vi "editConfiguration.vi"   [LabVIEW 2013]
uses:
  <userlib>/Common/ConfigurationEditor/ConfigurationEditor.lvclass
types:
  T1 = enum32{"Bad", "Idle", "Run top level", "Running"}
  T2 = enum32{"Invalid", "Standard", "Closed", "Hidden", "Minimized", "Maximized"}
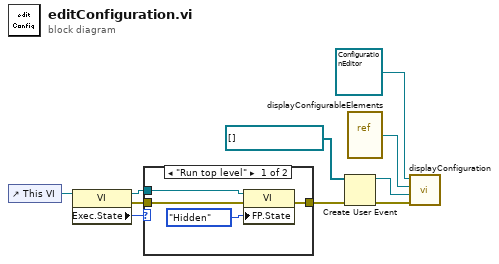
[diagram p0: block diagram]
diagram:
  n1 = control-ref of="This VI"() -> (w5:refnum<vi>)
  n2 = property class="VI"(reference=w5) -> (reference out=w3:refnum<vi>, error out=w1:errorcluster, "Exec.State"=w4:T1)  [unwired: 1 in]
  n3 = case shown="\"Run top level\"" w4 {
    tunnel: w3 -> [w13 _]
    tunnel: [w12 w15] -> w2
    tunnel: w1 -> [w11 w15]
    frame "Run top level" {
      n4 = property class="VI"(reference=w13, error in=w11, "FP.State"=T2."Hidden" ("Front Panel Window:State")) -> (error out=w12:errorcluster)  [unwired: 1 out]
    }
    frame "Running", Default {
    }
  }
  n5 = Create User Event(user event datatype=refnum<vi>[] [] ("cfgCtrlRefs"), error in=w2) -> (user event=w7:refnum<user-event>, error out=w6:errorcluster)
  n6 = vi-ref "displayConfigurableElements.vi"() -> (w10:refnum<vi>)
  n7 = call <userlib>:"displayConfiguration.vi"("error in (no error)"=w6, "ctrlRefArrayUsrEvnt"=w7, "configurableElementsVI"=w10, "ConfigurationEditor in"=refnum<class "ConfigurationEditor.lvclass"> refnum) -> ()  [unwired: 6 in, 2 out]
